vi "HooksRetractFull.vi"(10 "HooksInLimitSwitch":T1) -> (2 "Done?":bool)   [LabVIEW 2012]
uses:
  <vilib>/Rock Robotics/WPI/DigitalInput/WPI_DigitalInputDevRef.ctl
  <vilib>/Rock Robotics/SystemInterfaces/DIO/FPGA_DIOChannel.ctl
  <vilib>/Rock Robotics/SystemInterfaces/Typedef/FPGA_TypedefDigitalModule.ctl
  Robot Global Data.vi
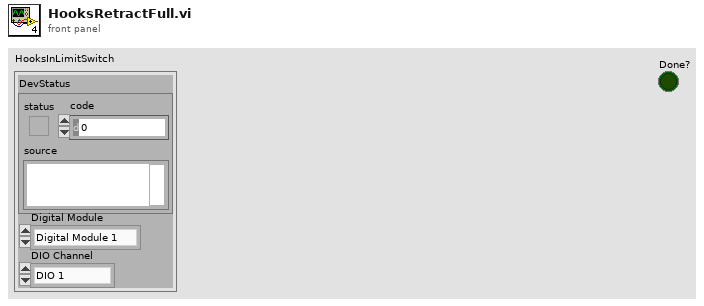
[diagram p1: front panel]
types:
  T1 = typedef "WPI_DigitalInputDevRef.ctl" = cluster{"DevStatus":errorcluster, "DIO Channel":T2, "Digital Module":T3}
  T2 = typedef "FPGA_DIOChannel.ctl" = enum8{"DIO 1", "DIO 2", "DIO 3", "DIO 4", "DIO 5", "DIO 6", "DIO 7", "DIO 8", "DIO 9", "DIO 10", "DIO 11", "DIO 12", "DIO 13", "DIO 14", "Invalid"}
  T3 = typedef "FPGA_TypedefDigitalModule.ctl" = enum16{"Digital Module 1", "Digital Module 2"}
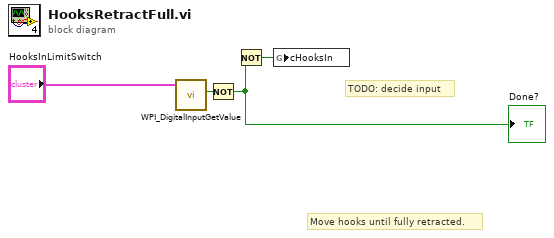
[diagram p0: block diagram]
diagram:
  # "Move hooks until fully retracted."
  # "TODO: decide input"
  n1 = call <vilib>:"WPI_DigitalInputGetValue.vi"("DigitalInputDevRef"="HooksInLimitSwitch") -> ("Value"=w3:bool)  [unwired: 8 in, 2 out]
  n2 = Not(x=w3) -> (.not. x?=w1:bool)
  "Done?" <- w1
  n3 = Not(x=w1) -> (.not. x?=w2:bool)
  n4 = global write "Robot Global Data.vi" "cHooksIn"(w2) -> ()
